vi "Reset Min-Max Pressure.vi"() -> (2 "Min Pressure Out":dbl, 3 "Max Pressure Out":dbl)   [LabVIEW 2020]
panel:
  in  "OK Button":bool
  in  "Min Pressure":dbl
  in  "Max Pressure":dbl min=-20.0 max=500.0
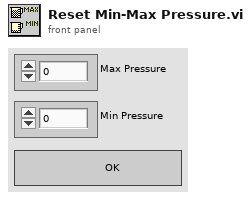
[diagram p1: front panel]
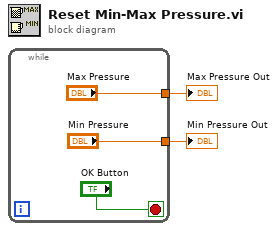
[diagram p0: block diagram]
diagram:
  n1 = while {
    tunnel: ["Max Pressure"] -> w1
    tunnel: ["Min Pressure"] -> w2
    stop <- "OK Button" stop-if-true
  }
  "Min Pressure Out" <- w2
  "Max Pressure Out" <- w1
